vi "Vision Research Phantom Series Self-Test.vi"(11 "Error In (no error)":errorcluster) -> (8 "Self-Test Error":u32, 10 "Self-Test Response":string, 15 "Error Out":errorcluster)   [LabVIEW 2013, in "VRI.lvlib"]
doc: "This VI returns a warning code because self test is not supported. This VI is included as part of the standard National Instruments driver requirements in case a self test feature is ever implemented.\n\nWritten by:\nBLOOMY CONTROLS, INC\nWINDSOR, CT 06095, USA\n860-298-9925\nwww.bloomy.com\nV1.0.0\nMay, 2004"
uses:
  VRI.lvlib
panel:
  # "For instructions on the use of this VI, press Ctrl+H to display the help window and move the mouse over the icon, controls, and indicators"
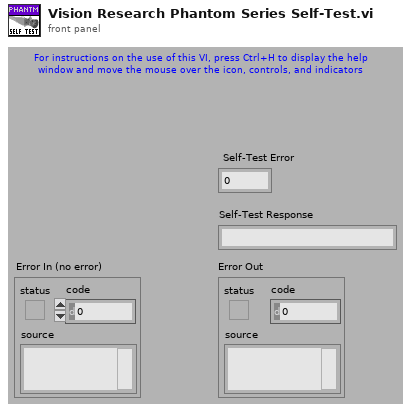
[diagram p1: front panel]
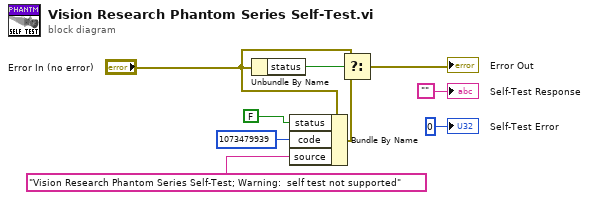
[diagram p0: block diagram]
diagram:
  n1 = Unbundle By Name("Error In (no error)") -> ("status"=w2:bool)
  n2 = Bundle By Name(cluster="Error In (no error)", "status"=FALSE, "code"=1073479939, "source"="Vision Research Phantom Series Self-Test; Warning:  self test not supported") -> (w1:errorcluster)
  n3 = Select(t="Error In (no error)", s=w2, f=w1) -> (s? t:f=→"Error Out":errorcluster)
  "Self-Test Response" <- ""
  "Self-Test Error" <- u32 0
